vi "FGV_PlotStyle.vi"(7 "Function":enum16{"Set", "Get"}(ring), 8 "error in (no error)":errorcluster, 10 "Input Cluster":T1={"BGColor"=0, "GridX"=FALSE, "GridY"=FALSE, "LineColorArray"=[0, 0, 0, 0, 0, 0, 0, 0, 0, 0], "LineWidthArray"=[0, 0, 0, 0, 0, 0, 0, 1, 0, 0]}) -> (0 "error out":errorcluster, 2 "Output Cluster":T1)   [LabVIEW 2018]
uses:
  Ctl/RegistyFunc.ctl
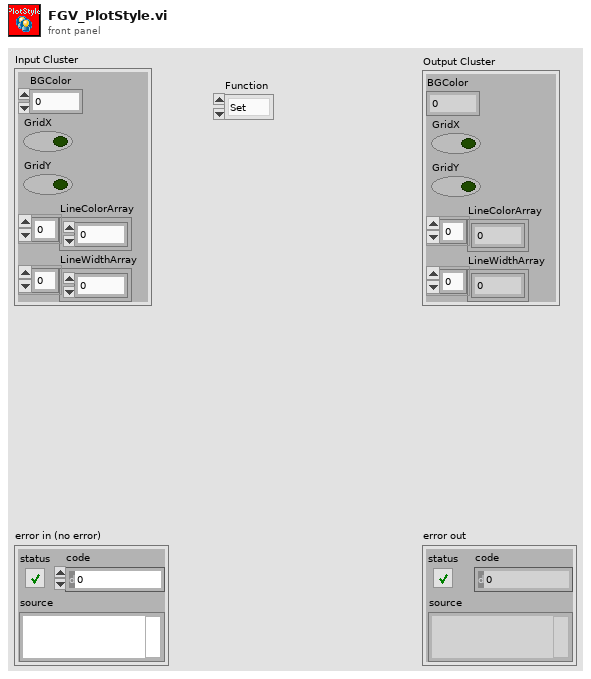
[diagram p1: front panel]
types:
  T1 = cluster{"BGColor":u32, "GridX":bool, "GridY":bool, "LineColorArray":u32[], "LineWidthArray":u8[]}
  T2 = typedef "RegistyFunc.ctl" = enum16{"None", "FileAutoSave", "FileNoise", "FileSN", "ExeStatu", "WorkFolderPath", "MethodPath", "AVGItem", "LoopItem", "AutoRun", "BGColor", "LineColor", "LineWidth", "XGrid", "YGrid", "DeviceRefnum"}
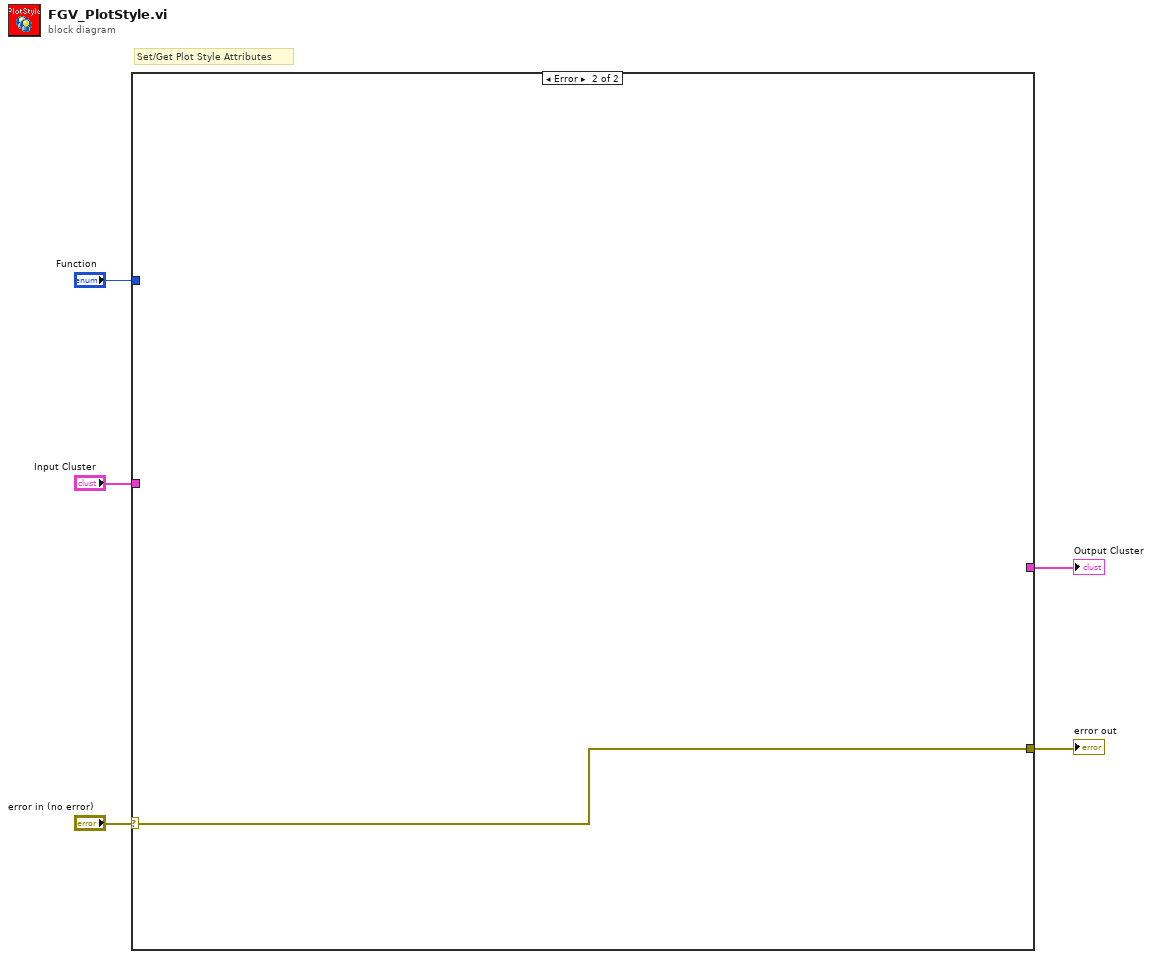
[diagram p0: block diagram]
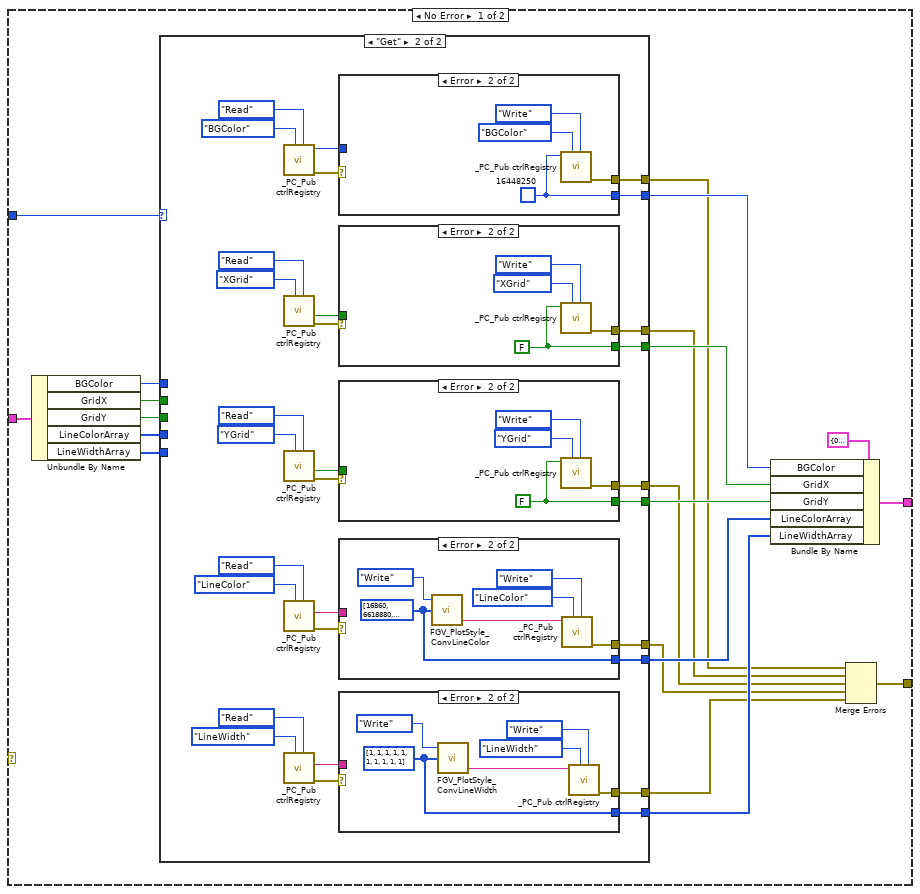
[diagram p2: hidden frame]
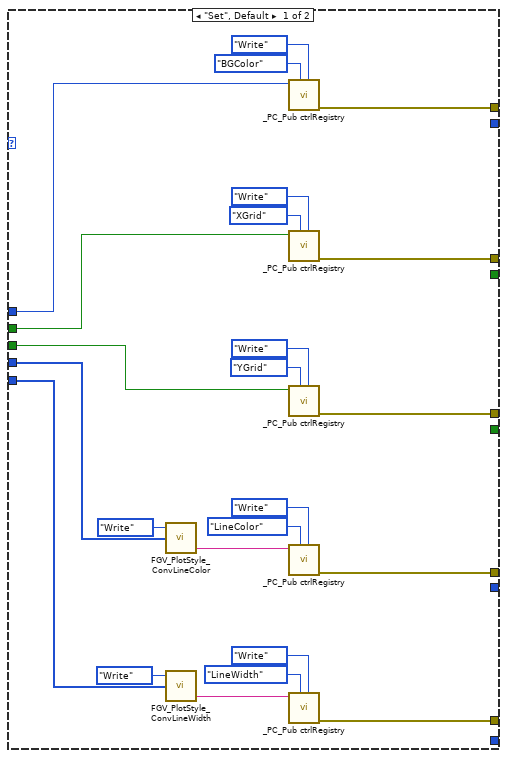
[diagram p3: hidden frame]
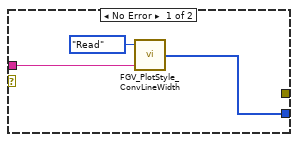
[diagram p7: hidden frame]
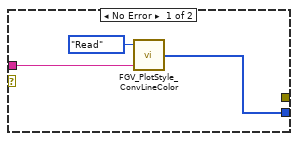
[diagram p8: hidden frame]
diagram:
  # "Set/Get Plot Style Attributes"
  n1 = case shown="Error" "error in (no error)" {
    selector: "error in (no error)" -> [_ w113]
    tunnel: "Function" -> [w25 _]
    tunnel: "Input Cluster" -> [w24 _]
    tunnel: [w14 _] -> w3
    tunnel: [w6 w113] -> w1
    frame No Error {
      n2 = Unbundle By Name(w24) -> ("BGColor"=w23:u32, "GridX"=w22:bool, "GridY"=w21:bool, "LineColorArray"=w20:u32[], "LineWidthArray"=w19:u8[])
      n3 = case shown="\"Get\"" w25 {
        tunnel: w23 -> [w38 _]
        tunnel: w22 -> [w39 _]
        tunnel: w21 -> [w26 _]
        tunnel: w20 -> [w35 _]
        tunnel: w19 -> [w33 _]
        tunnel: [_ w55] -> w15
        tunnel: [_ w56] -> w16
        tunnel: [_ w63] -> w17
        tunnel: [_ w68] -> w13
        tunnel: [_ w66] -> w12
        tunnel: [w28 w54] -> w11
        tunnel: [w27 w53] -> w10
        tunnel: [w29 w52] -> w9
        tunnel: [w30 w51] -> w8
        tunnel: [w31 w50] -> w7
        frame "Set", Default {
          n4 = call "FGV_PlotStyle_ConvLineColor.vi"("LineColorArray"=w35, "Func"=enum16{"Write", "Read"}."Write") -> ("spreadsheet string"=w36:string)  [unwired: 2 in, 1 out]
          n5 = call "FGV_PlotStyle_ConvLineWidth.vi"("LineWidthArray"=w33, "Func"=enum16{"Write", "Read"}."Write") -> ("spreadsheet string"=w32:string)  [unwired: 2 in, 1 out]
          n6 = call "_PC_Pub ctrlRegistry.vi"("type"=enum16{"None", "Write", "Read"}."Write", "function"=RegistyFunc."BGColor", "write value"=w38) -> ("error out"=w28:errorcluster)  [unwired: 5 in, 3 out]
          n7 = call "_PC_Pub ctrlRegistry.vi"("type"=enum16{"None", "Write", "Read"}."Write", "function"=RegistyFunc."XGrid", "write value"=w39) -> ("error out"=w27:errorcluster)  [unwired: 5 in, 3 out]
          n8 = call "_PC_Pub ctrlRegistry.vi"("type"=enum16{"None", "Write", "Read"}."Write", "function"=RegistyFunc."YGrid", "write value"=w26) -> ("error out"=w29:errorcluster)  [unwired: 5 in, 3 out]
          n9 = call "_PC_Pub ctrlRegistry.vi"("type"=enum16{"None", "Write", "Read"}."Write", "function"=RegistyFunc."LineColor", "write value"=w36) -> ("error out"=w30:errorcluster)  [unwired: 5 in, 3 out]
          n10 = call "_PC_Pub ctrlRegistry.vi"("type"=enum16{"None", "Write", "Read"}."Write", "function"=RegistyFunc."LineWidth", "write value"=w32) -> ("error out"=w31:errorcluster)  [unwired: 5 in, 3 out]
        }
        frame "Get" {
          n11 = call "_PC_Pub ctrlRegistry.vi"("type"=enum16{"None", "Write", "Read"}."Read", "function"=RegistyFunc."BGColor") -> ("error out"=w64:errorcluster, "DWORD outpur"=w65:u32)  [unwired: 6 in, 2 out]
          n12 = call "_PC_Pub ctrlRegistry.vi"("type"=enum16{"None", "Write", "Read"}."Read", "function"=RegistyFunc."XGrid") -> ("error out"=w60:errorcluster, "Boolean output"=w59:bool)  [unwired: 6 in, 2 out]
          n13 = call "_PC_Pub ctrlRegistry.vi"("type"=enum16{"None", "Write", "Read"}."Read", "function"=RegistyFunc."YGrid") -> ("error out"=w57:errorcluster, "Boolean output"=w58:bool)  [unwired: 6 in, 2 out]
          n14 = call "_PC_Pub ctrlRegistry.vi"("type"=enum16{"None", "Write", "Read"}."Read", "function"=RegistyFunc."LineColor") -> ("error out"=w62:errorcluster, "SZ output"=w69:string)  [unwired: 6 in, 2 out]
          n15 = call "_PC_Pub ctrlRegistry.vi"("type"=enum16{"None", "Write", "Read"}."Read", "function"=RegistyFunc."LineWidth") -> ("error out"=w61:errorcluster, "SZ output"=w67:string)  [unwired: 6 in, 2 out]
          n16 = case shown="Error" w64 {
            tunnel: w65 -> [w90 _]
            tunnel: [w90 w92] -> w63
            tunnel: [_ w91] -> w54
            frame No Error {
            }
            frame Error {
              w92 = u32 16448250
              n17 = call "_PC_Pub ctrlRegistry.vi"("type"=enum16{"None", "Write", "Read"}."Write", "function"=RegistyFunc."BGColor", "write value"=w92) -> ("error out"=w91:errorcluster)  [unwired: 5 in, 3 out]
            }
          }
          n18 = case shown="Error" w60 {
            tunnel: [w85 w87] -> w56
            tunnel: w59 -> [w85 _]
            tunnel: [_ w86] -> w53
            frame No Error {
            }
            frame Error {
              w87 = FALSE
              n19 = call "_PC_Pub ctrlRegistry.vi"("type"=enum16{"None", "Write", "Read"}."Write", "function"=RegistyFunc."XGrid", "write value"=w87) -> ("error out"=w86:errorcluster)  [unwired: 5 in, 3 out]
            }
          }
          n20 = case shown="Error" w57 {
            tunnel: [w80 w82] -> w55
            tunnel: w58 -> [w80 _]
            tunnel: [_ w81] -> w52
            frame No Error {
            }
            frame Error {
              w82 = FALSE
              n21 = call "_PC_Pub ctrlRegistry.vi"("type"=enum16{"None", "Write", "Read"}."Write", "function"=RegistyFunc."YGrid", "write value"=w82) -> ("error out"=w81:errorcluster)  [unwired: 5 in, 3 out]
            }
          }
          n22 = case shown="Error" w62 {
            tunnel: w69 -> [w105 _]
            tunnel: [w104 w108] -> w68
            tunnel: [_ w107] -> w51
            frame No Error {
              n23 = call "FGV_PlotStyle_ConvLineColor.vi"("spreadsheet string"=w105, "Func"=enum16{"Write", "Read"}."Read") -> ("LineColorArray"=w104:u32[])  [unwired: 2 in, 1 out]
            }
            frame Error {
              w108 = u32[] [16860, 6618880, 16711680, 8404992, 9567230, 16776960, 4194304, 15425504, 11377477, 4227200]
              n24 = call "FGV_PlotStyle_ConvLineColor.vi"("LineColorArray"=w108, "Func"=enum16{"Write", "Read"}."Write") -> ("spreadsheet string"=w112:string)  [unwired: 2 in, 1 out]
              n25 = call "_PC_Pub ctrlRegistry.vi"("type"=enum16{"None", "Write", "Read"}."Write", "function"=RegistyFunc."LineColor", "write value"=w112) -> ("error out"=w107:errorcluster)  [unwired: 5 in, 3 out]
            }
          }
          n26 = case shown="Error" w61 {
            tunnel: [w95 w99] -> w66
            tunnel: w67 -> [w97 _]
            tunnel: [_ w98] -> w50
            frame No Error {
              n27 = call "FGV_PlotStyle_ConvLineWidth.vi"("spreadsheet string"=w97, "Func"=enum16{"Write", "Read"}."Read") -> ("LineWidthArray"=w95:u8[])  [unwired: 2 in, 1 out]
            }
            frame Error {
              w99 = u8[] [1, 1, 1, 1, 1, 1, 1, 1, 1, 1]
              n28 = call "FGV_PlotStyle_ConvLineWidth.vi"("LineWidthArray"=w99, "Func"=enum16{"Write", "Read"}."Write") -> ("spreadsheet string"=w103:string)  [unwired: 2 in, 1 out]
              n29 = call "_PC_Pub ctrlRegistry.vi"("type"=enum16{"None", "Write", "Read"}."Write", "function"=RegistyFunc."LineWidth", "write value"=w103) -> ("error out"=w98:errorcluster)  [unwired: 5 in, 3 out]
            }
          }
        }
      }
      n30 = Bundle By Name(cluster=T1 {"BGColor"=0, "GridX"=FALSE, "GridY"=FALSE, "LineColorArray"=[0, 0, 0, 0, 0, 0, 0, 0, 0, 0], "LineWidthArray"=[0, 0, 0, 0, 0, 0, 0, 0, 0, 0]} ("Output Cluster"), "BGColor"=w17, "GridX"=w16, "GridY"=w15, "LineColorArray"=w13, "LineWidthArray"=w12) -> (w14:T1)
      n31 = Merge Errors(w11, w10, w9, w8, w7) -> (w6:errorcluster)
    }
    frame Error {
    }
  }
  "Output Cluster" <- w3
  "error out" <- w1
